vi "LIN EX Master Get Sch.vi"(9 "pLINMsg":T1, 10 "LINIndex":u8, 11 "DevHandle":i32) -> (1 "pLINMsg out":T1, 3 "function return":i32)   [LabVIEW 2010, in "usb2lin_ex.lvlib"]
doc: "int WINAPI LIN_EX_MasterGetSch(int DevHandle,unsigned char LINIndex,LIN_EX_MSG *pLINMsg);"
uses:
  usb2lin_ex.lvlib
  USB2XXX.dll
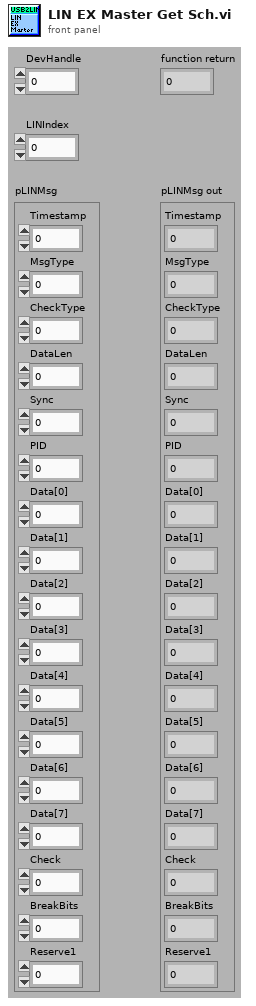
[diagram p1: front panel]
types:
  T1 = cluster{"Timestamp":u32, "MsgType":u8, "CheckType":u8, "DataLen":u8, "Sync":u8, "PID":u8, "Data[0]":u8, "Data[1]":u8, "Data[2]":u8, "Data[3]":u8, "Data[4]":u8, "Data[5]":u8, "Data[6]":u8, "Data[7]":u8, "Check":u8, "BreakBits":u8, "Reserve1":u8}
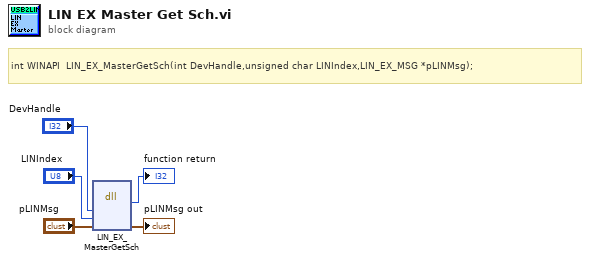
[diagram p0: block diagram]
diagram:
  # "int WINAPI  LIN_EX_MasterGetSch(int DevHandle,unsigned char LINIndex,LIN_EX_MSG *pLINMsg);"
  n1 = dll-call lib="E:/OtherWork/STM32/USB2XXX_Example/trunk/SDK/api/Labview/USB2XXX.*" fn="LIN_EX_MasterGetSch"("DevHandle"="DevHandle", "LINIndex"="LINIndex", "pLINMsg"="pLINMsg") -> (→"function return":i32, "pLINMsg"=→"pLINMsg out":T1)  [unwired: 5 in, 2 out]
